vi "Init.vi"(8 "error in (no error)":errorcluster, 11 "Config File":path) -> (0 "error out":errorcluster)   [LabVIEW 2016, in "Log4Lv.lvlib"]
doc: "Use this template to build a VI to use as a subVI."
uses:
  Log4Lv.lvlib
  Private/Config Global.vi
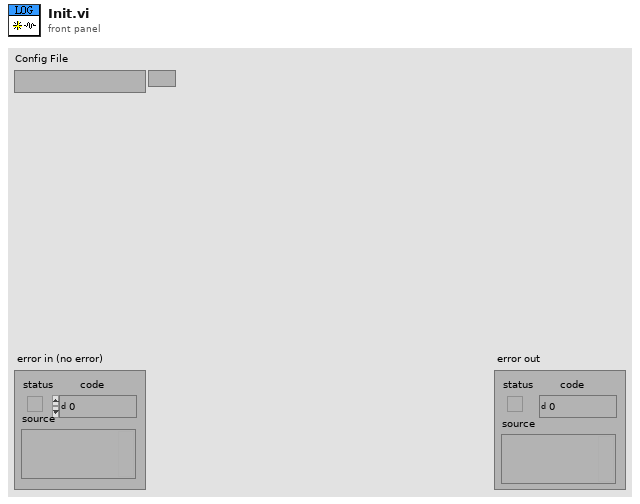
[diagram p1: front panel]
types:
  T1 = cluster{"LogName":string, "Level":enum16{"Disable", "Error", "Warn", "Info", "Debug"}, "LogFolder":path, "MaxFileSize":i32, "FileExtension":string, "TimeSytle":string, "LogStyle":string}
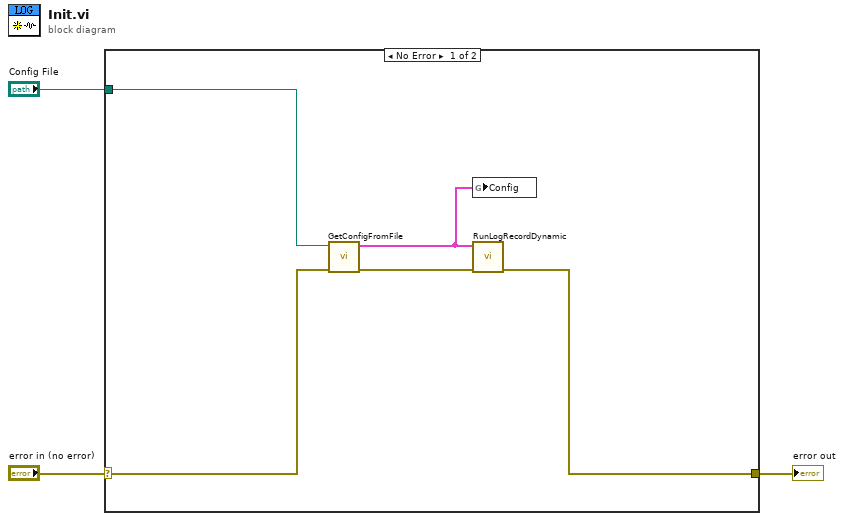
[diagram p0: block diagram]
diagram:
  n1 = case shown="No Error" "error in (no error)" {
    selector: "error in (no error)" -> [w7 w9]
    tunnel: [w5 w9] -> w2
    tunnel: "Config File" -> [w8 _]
    frame No Error {
      n2 = call "GetConfigFromFile.vi"("error in (no error)"=w7, "Config File"=w8) -> ("error out"=w6:errorcluster, "Config"=w4:T1)  [unwired: 8 in]
      n3 = global write "Config Global.vi" "Config"(w4) -> ()
      n4 = call "RunLogRecordDynamic.vi"("error in (no error)"=w6, "Config"=w4) -> ("error out"=w5:errorcluster)  [unwired: 9 in]
    }
    frame Error {
    }
  }
  "error out" <- w2
